vi "ApplyConfigQueued.vi"(8 "error in":errorcluster, 10 "UpdatedChannel.lvclass":refnum<class "T560Channel.lvclass">, 11 "T560Session in":refnum<class "T560Session.lvclass">) -> (0 "error out":errorcluster, 3 "T560Session out":refnum<class "T560Session.lvclass">)   [LabVIEW 2020, in "T560Session.lvclass"]
doc: "Send the channels configuration to the physical device, to be applied at the end of the timing cycle"
uses:
  T560Session.lvclass
  T560Channel.lvclass
  T560Session.lvclass/T560Session.ctl
panel:
  out "Array":string[](array[string])
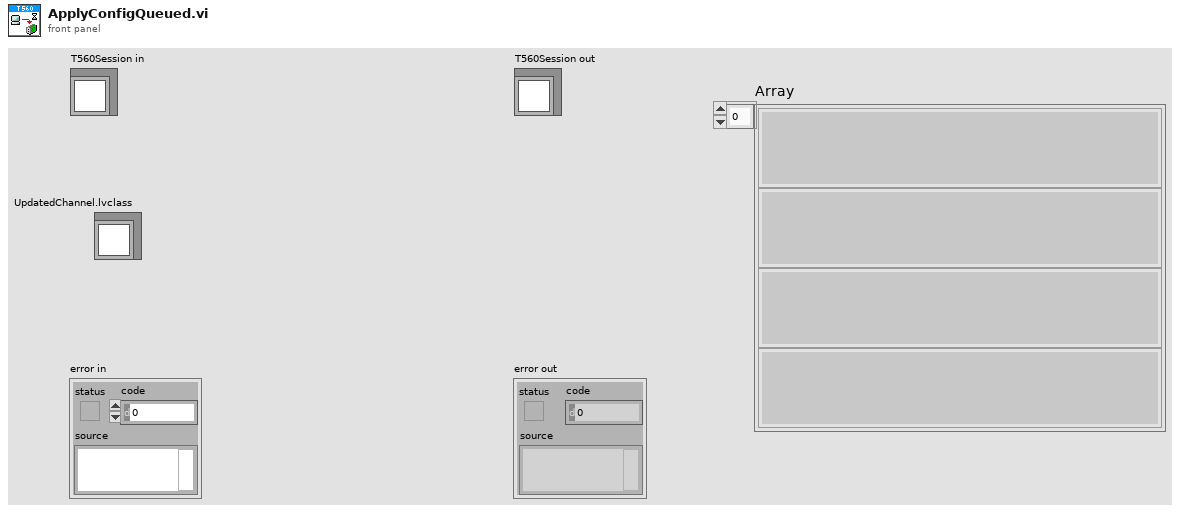
[diagram p1: front panel]
types:
  T1 = typedef "T560Channel.lvclass/ChannelName.ctl" = enum16{"Null", "A", "B", "C", "D", "Trigger"}
  T2 = typedef "Highlandt564.lvlib/T560Channel.lvclass/ChannelName.ctl" = enum16{"Null", "A", "B", "C", "D", "Trigger"}
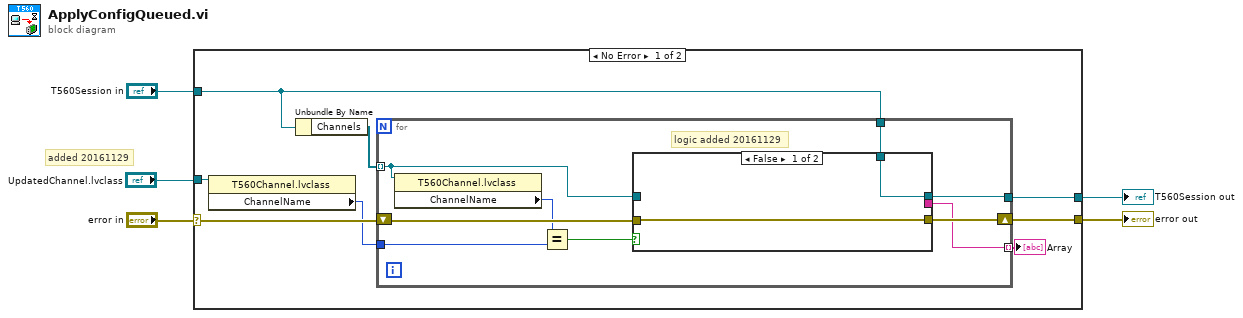
[diagram p0: block diagram]
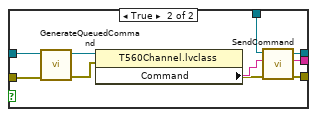
[diagram p2: hidden frame]
diagram:
  # "added 20161129"
  n1 = case shown="No Error" "error in" {
    selector: "error in" -> [w13 w36]
    tunnel: [w12 w36] -> w4
    tunnel: [w10 w35] -> w2
    tunnel: "T560Session in" -> [w11 w35]
    tunnel: "UpdatedChannel.lvclass" -> [w7 _]
    frame No Error {
      n2 = property class="T560Channel.lvclass"(reference=w7) -> ("ChannelName"=w6:T1)  [unwired: 1 in, 2 out]
      n3 = Unbundle By Name(w11) -> ("Channels"=w8:refnum<class "T560Channel.lvclass">[])
      n4 = for {
        tunnel: w8 -> [w17] mode=indexing
        tunnel: w11 -> [w21]
        shift-right: [w20] -> w12
        shift-left: w13 -> [w22]
        tunnel: [w19] -> w10
        tunnel: [w18] -> w9 mode=indexing
        tunnel: w6 -> [w15]
        # "logic added 20161129"
        n5 = property class="T560Channel.lvclass"(reference=w17) -> ("ChannelName"=w16:T2)  [unwired: 1 in, 2 out]
        n6 = Equal?(x=w16, y=w15) -> (x = y?=w14:bool)
        n7 = case shown="False" w14 {
          tunnel: w22 -> [w23 w34]
          tunnel: w21 -> [w24 w29]
          tunnel: [w23 w28] -> w20
          tunnel: [w24 w27] -> w19
          tunnel: [_ w26] -> w18
          tunnel: w17 -> [_ w25]
          frame False {
          }
          frame True {
            n8 = call-dynamic "GenerateQueuedCommand.vi"("error in"=w34, "T560Object in"=w25) -> ("error out"=w32:errorcluster, "T560Object out"=w33:refnum<class "T560Channel.lvclass">)  [unwired: 8 in]
            n9 = property class="T560Channel.lvclass"(reference=w33, error in=w32) -> (error out=w30:errorcluster, "Command"=w31:string)  [unwired: 1 out]
            n10 = call-dynamic "SendCommand.vi"("error in"=w30, "Command"=w31, "T560Session in"=w29) -> ("error out"=w28:errorcluster, "Response"=w26:string, "T560Session out"=w27:refnum<class "T560Session.lvclass">)  [unwired: 6 in]
          }
        }
      }
      "Array" <- w9
    }
    frame Error {
    }
  }
  "error out" <- w4
  "T560Session out" <- w2
